vi "Servo Camera.vi"() -> ()   [LabVIEW 2013]
doc: "<B>Servo Camera Example</B> will track a colored object by moving a gimbal mounted camera to keep the object centered in the image. It assumes the camera is mounted upright, and that the DS is connected. It is written to control two servos, but will work fine with one. To tune the colors, you may find it easiest to set the Operation control to Camera Display. This way the servos will not update and you can experiment with the colors to get a good mask.\nOnce the color thresholds are set appropriately for the object you are tracking, switch Operation to GimbalTrack."
uses:
  <vilib>/addons/control/pid/pid.llb/PID Control Input Filter (DBL).vi
  <vilib>/Rock Robotics/WPI/Camera/WPI_CameraFrameRate.ctl
  <vilib>/Rock Robotics/WPI/Camera/WPI_CameraImageSize.ctl
  Control States.ctl
  <vilib>/Rock Robotics/SystemInterfaces/DIO/FPGA_DIOPWMChannel.ctl
panel:
  in  "stop":bool
  in  "Operation":enum32{"Camera Display", "Gimbal Track"}(radio)
  out "Servo Tracking State":T2
  in  "Servo Positions":cluster{"X":dbl, "Y":dbl}={"X"=85.52840986947938, "Y"=85.0} {"Y" scale=0.0..170.0; "X" scale=0.0..170.0}
  in  "Y Channel":T3=enum."PWM 2"
  in  "Loop Sleep":u32=20
  in  "Loop Sleep":u32=80
  in  "X Channel":T3
  in  "Image Decimation":cluster{"X":dbl, "Y":dbl}={"X"=5.0, "Y"=4.0}
  in  "Color Ranges":T4={"Hue"={"Min"=55, "Max"=93}, "Sat"={"Min"=41, "Max"=255}, "Luma"={"Min"=64, "Max"=255}}
  in  "Smooth":bool=TRUE
  out "Mask after threshold":T5(plugin-control)
  in  "Display Mask":bool=TRUE
  out "Camera Image":T5(plugin-control)
  # "This example will track a colored object by moving a gimbal mounted camera to keep the object centered in the image. It assumes the camera is mounted upright, and that the DS is connected. It is written to control two servos, but will work fine with one. To tune the colors, you may find it easiest to set the Operation control to Camera Display. This way the servos will not update and you can experiment with the colors to get a good mask.\nOnce the color thresholds are set appropriately for the object you are tracking, switch Operation to GimbalTrack."
  # "Servo Settings"
  # "Camera Settings"
  # "Hues are ~ 70, 150, and 250\nfor Green, Blue, and Red."
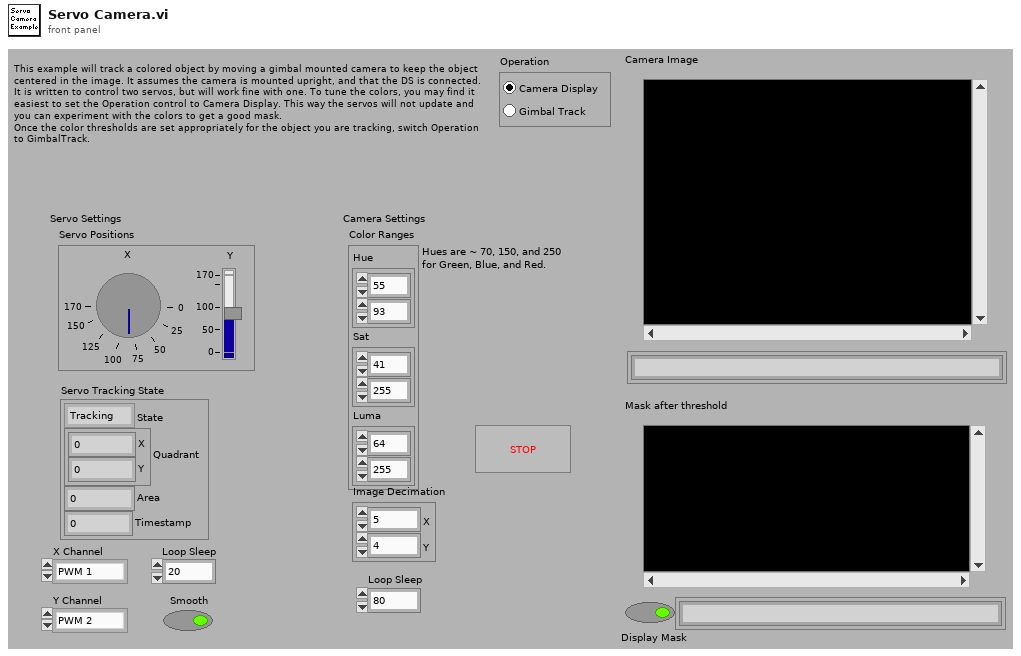
[diagram p1: front panel]
types:
  T1 = typedef "Control States.ctl" = enum16{"Tracking", "Lost Small", "Lost-Patience", "Search-Begin", "Searching", "Lost - Edge"}
  T2 = cluster{"State":T1, "Quadrant":cluster{"X":i32, "Y":i32}, "Area":i32, "Timestamp":u32}
  T3 = typedef "FPGA_DIOPWMChannel.ctl" = enum8{"PWM 1", "PWM 2", "PWM 3", "PWM 4", "PWM 5", "PWM 6", "PWM 7", "PWM 8", "PWM 9", "PWM 10", "Invalid"}
  T4 = cluster{"Hue":cluster{"Min":i32, "Max":i32}, "Sat":cluster{"Min":i32, "Max":i32}, "Luma":cluster{"Min":i32, "Max":i32}}
  T5 = typedef "IMAQ Image.ctl" = refnum<image>
  T6 = typedef "WPI_CameraImageSize.ctl" = enum16{"640x480", "320x240", "160x120"}
  T7 = typedef "WPI_CameraFrameRate.ctl" = u32
  T8 = typedef "WPI_CameraDevRef.ctl" = cluster{"Camera Address":string, "CameraStatus":errorcluster, "Acquire Image Notifier":refnum<notifier>}
  T9 = typedef "WPI_ServoDeviceRef.ctl" = cluster{"DeviceStatus":errorcluster, "Digital Module":T10, "PWM Channel":T3, "DeadBand":T11}
  T10 = typedef "FPGA_TypedefDigitalModule.ctl" = enum16{"Digital Module 1", "Digital Module 2"}
  T11 = typedef "WPI_PWMDeadband.ctl" = cluster{"Name":string, "maxPositivePwm":i32, "minPositivePwm":i32, "centerPwm":i32, "maxNegativePwm":i32, "minNegativePwm":i32, "angularRange":u16}
  T12 = cluster{"Left":i32, "Top":i32, "Right":i32, "Bottom":i32}
  T13 = cluster{"State":T1, "Quadrant":cluster{"X":i32, "Y":i32}, "Area":i32, "millisecond timer value":u32}
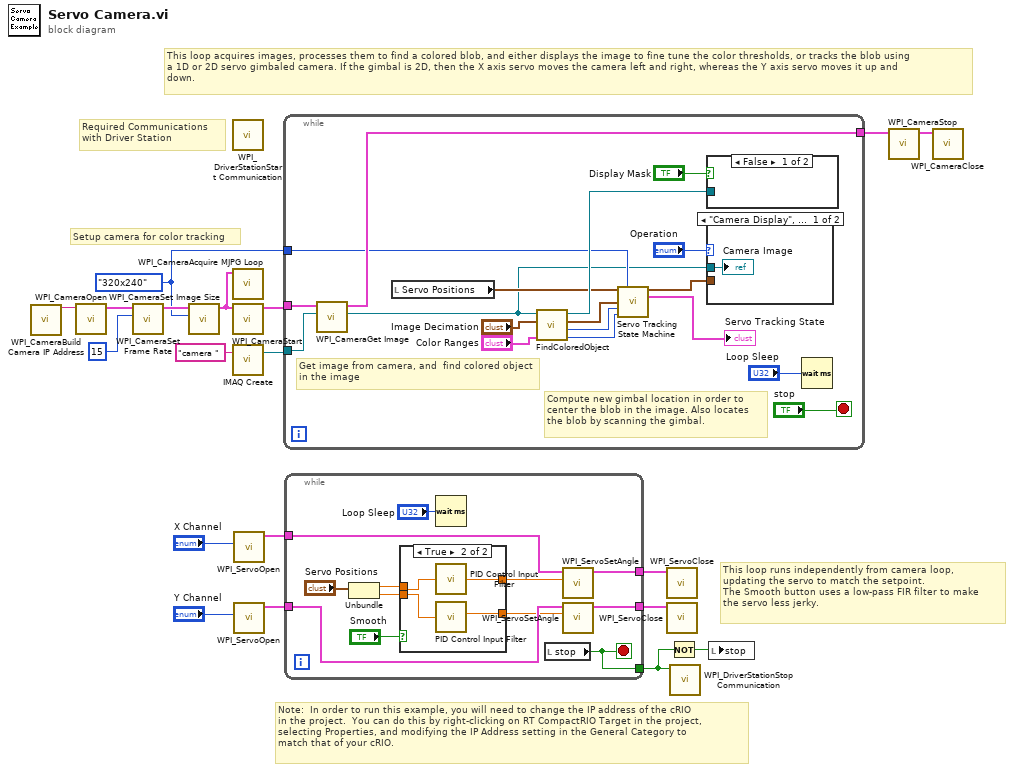
[diagram p0: block diagram]
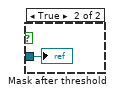
[diagram p2: hidden frame]
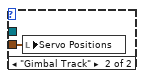
[diagram p3: hidden frame]
diagram:
  w7 = WPI_CameraImageSize."320x240" ("Image Size")
  # "Note:  In order to run this example, you will need to change the IP address of the cRIO\nin the project.  You can do this by right-clicking on RT CompactRIO Target in the project,\nselecting Properties, and modifying the IP Address setting in the General Category to \nmatch that of your cRIO."
  # "This loop acquires images, processes them to find a colored blob, and either displays the image to fine tune the color thresholds, or tracks the blob using\na 1D or 2D servo gimbaled camera. If the gimbal is 2D, then the X axis servo moves the camera left and right, whereas the Y axis servo moves it up and\ndown."
  # "This loop runs independently from camera loop,\nupdating the servo to match the setpoint.\nThe Smooth button uses a low-pass FIR filter to make\nthe servo less jerky."
  # "Setup camera for color tracking"
  # "Required Communications\nwith Driver Station"
  n1 = call <vilib>:"WPI_CameraBuild Camera IP Address.vi"() -> ("Camera Address"=w4:string)  [unwired: 11 in]
  n2 = call <vilib>:"WPI_CameraOpen.vi"("Camera Address"=w4) -> ("CameraDevRef"=w8:T8)  [unwired: 1 in, 9 out]
  n3 = call <vilib>:"WPI_CameraSet Frame Rate.vi"("Frame Rate (fps)"=T7 15, "CameraDevRef"=w8) -> ("CameraDevRef Out"=w9:T8)  [unwired: 1 in, 8 out]
  n4 = call <vilib>:"WPI_CameraSet Image Size.vi"("Image Size"=w7, "CameraDevRef"=w9) -> ("CameraDevRef Out"=w3:T8)  [unwired: 1 in, 8 out]
  n5 = call <vilib>:"WPI_DriverStationStart Communication.vi"() -> ()  [unwired: 1 in, 11 out]
  n6 = call <vilib>:"WPI_CameraAcquire MJPG Loop.vi"("CameraDevRef"=w3) -> ()  [unwired: 11 in]
  n7 = call <vilib>:"WPI_CameraStart.vi"("CameraDevRef"=w3) -> ("CameraDevRef Out"=w12:T8)  [unwired: 1 in, 9 out]
  n8 = call "IMAQ Create"("Image Name"="camera ") -> ("New Image"=w13:T5)  [unwired: 3 in, 2 out]
  n9 = call <vilib>:"WPI_ServoOpen.vi"("PWM Channel"="X Channel") -> ("ServoDeviceRef"=w17:T9)  [unwired: 3 in, 7 out]
  n10 = call <vilib>:"WPI_ServoOpen.vi"("PWM Channel"="Y Channel") -> ("ServoDeviceRef"=w16:T9)  [unwired: 3 in, 7 out]
  n11 = while {
    tunnel: w12 -> [w31]
    tunnel: [w30] -> w11
    tunnel: w13 -> [w36]
    tunnel: w7 -> [w27]
    stop <- "stop" stop-if-true
    # "Compute new gimbal location in order to\ncenter the blob in the image. Also locates\nthe blob by scanning the gimbal."
    # "Get image from camera, and  find colored object in the image"
    n12 = call <vilib>:"WPI_CameraGet Image.vi"("Image"=w36, "CameraDevRef"=w31) -> ("Image Out"=w23:T5, "CameraDevRef Out"=w30:T8)  [unwired: 1 in, 7 out]
    n13 = local read "Servo Positions"() -> (w28:cluster{"X":dbl, "Y":dbl})
    n14 = call "FindColoredObject.vi"("Color Range"="Color Ranges", "Decimate by"="Image Decimation", "Color Image In"=w23) -> ("Area"=w21:i32, "Particles"=w25:i32, "Rectangle"=w26:T12, "Mask Image"=w29:T5)  [unwired: 3 out]
    n15 = call "Servo Tracking State Machine.vi"("Servo Positions In"=w28, "Image Size"=w27, "Rectangle"=w26, "Particles"=w25, "Area"=w21) -> ("Servo Positions"=w34:cluster{"X":dbl, "Y":dbl}, "Tracking State Info"=→"Servo Tracking State":T13)  [unwired: 2 in, 7 out]
    n16 = case shown="False" "Display Mask" {
      tunnel: w29 -> [_ w38]
      frame False {
      }
      frame True {
        "Mask after threshold" <- w38
      }
    }
    n17 = case shown="\"Camera Display\", Default" "Operation" {
      tunnel: w34 -> [_ w40]
      tunnel: w23 -> [w39 _]
      frame "Camera Display", Default {
        "Camera Image" <- w39
      }
      frame "Gimbal Track" {
        n18 = local write "Servo Positions"(w40) -> ()
      }
    }
    n19 = Wait (ms)(milliseconds to wait="Loop Sleep") -> ()  [unwired: 1 out]
  }
  n20 = while {
    tunnel: w17 -> [w50]
    tunnel: [w52] -> w6
    tunnel: w16 -> [w49]
    tunnel: [w48] -> w5
    tunnel: [w41] -> w2
    stop <- w41 stop-if-true
    n21 = Unbundle("Servo Positions") -> ("X"=w46:dbl, "Y"=w44:dbl)
    n22 = case shown="True" "Smooth" {
      tunnel: w46 -> [w54 w58]
      tunnel: [w54 w57] -> w45
      tunnel: w44 -> [w53 w56]
      tunnel: [w53 w55] -> w43
      frame False {
      }
      frame True {
        n23 = call-poly <vilib>:"PID Control Input Filter.vi"("input"=w58) -> ("output"=w57:dbl)  [unwired: 1 in, 3 out]
        n24 = call-poly <vilib>:"PID Control Input Filter.vi"("input"=w56) -> ("output"=w55:dbl)  [unwired: 1 in, 3 out]
      }
    }
    n25 = Wait (ms)(milliseconds to wait="Loop Sleep") -> ()  [unwired: 1 out]
    n26 = local read "stop"() -> (w41:bool)
    n27 = call <vilib>:"WPI_ServoSetAngle.vi"("Angle"=w45, "ServoDeviceRef"=w50) -> ("ServoDeviceRef"=w52:T9)  [unwired: 1 in, 8 out]
    n28 = call <vilib>:"WPI_ServoSetAngle.vi"("Angle"=w43, "ServoDeviceRef"=w49) -> ("ServoDeviceRef"=w48:T9)  [unwired: 1 in, 8 out]
  }
  n29 = call <vilib>:"WPI_ServoClose.vi"("MotorControlDevRef"=w6) -> ()  [unwired: 1 in, 10 out]
  n30 = call <vilib>:"WPI_ServoClose.vi"("MotorControlDevRef"=w5) -> ()  [unwired: 1 in, 10 out]
  n31 = Not(x=w2) -> (.not. x?=w1:bool)
  n32 = call <vilib>:"WPI_DriverStationStop Communication.vi"("StopCommunication"=w2) -> ()  [unwired: 1 in, 10 out]
  n33 = local write "stop"(w1) -> ()
  n34 = call <vilib>:"WPI_CameraStop.vi"("CameraDevRef"=w11) -> ("CameraDevRef Out"=w15:T8)  [unwired: 1 in, 9 out]
  n35 = call <vilib>:"WPI_CameraClose.vi"("CameraDevRef"=w15) -> ()  [unwired: 1 in, 10 out]
